vi "Convert Relative to Absolute Project Paths.vi"(9 "VI Relative Paths":string[](array[string]), 10 "Project File":path) -> (2 "VI Absolute Paths":path[](array[path]))   [LabVIEW 2011, in "VITesterUtilities.lvlib"]
uses:
  Libraries/VITesterUtilities.lvlib
  <userlib>/_OpenG.lib/file/file.llb/Build Path - File Names Array - path__ogtk.vi
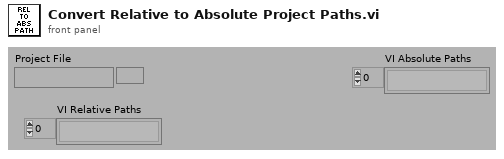
[diagram p1: front panel]
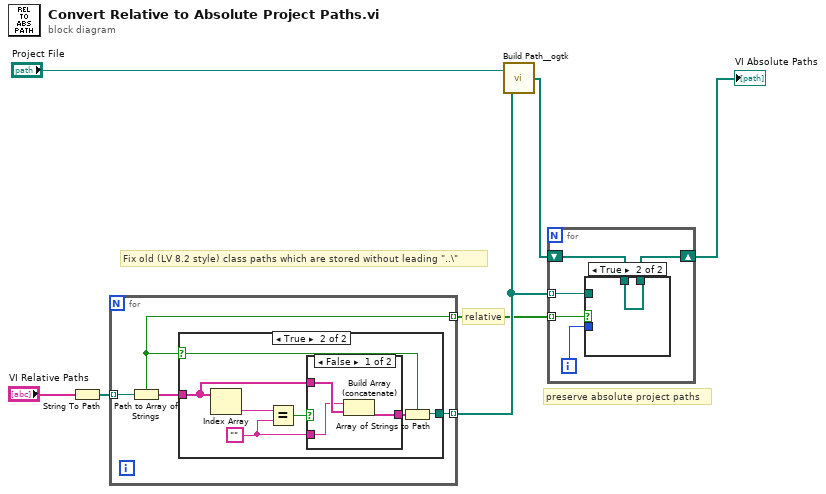
[diagram p0: block diagram]
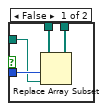
[diagram p2: hidden frame]
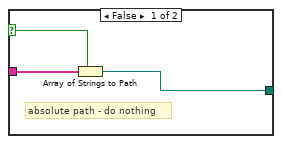
[diagram p3: hidden frame]
diagram:
  # "Fix old (LV 8.2 style) class paths which are stored without leading \"..\\\""
  # "preserve absolute project paths"
  # "relative"
  n1 = String To Path(string="VI Relative Paths") -> (path=w3:path[])
  n2 = for {
    tunnel: w3 -> [w11] mode=indexing
    tunnel: [w9] -> w7 mode=indexing
    tunnel: [w8] -> w4 mode=indexing
    n3 = Path to Array of Strings(0:w11) -> (1:w8:bool, 2:w10:string[])
    n4 = case shown="True" w8 {
      selector: w8 -> [w14 w16]
      tunnel: w10 -> [w13 w19]
      tunnel: [w12 w18] -> w9
      frame False {
        # "absolute path - do nothing"
        n5 = Array of Strings to Path(0:w13, 1:w14) -> (2:w12:path)
      }
      frame True {
        w15 = ""
        n6 = Index Array(array=w19) -> (element=w21:string)  [unwired: 1 in]
        n7 = Equal?(x=w21, y=w15) -> (x = y?=w20:bool)
        n8 = case shown="False" w20 {
          tunnel: w19 -> [w24 w25]
          tunnel: w15 -> [w23 _]
          tunnel: [w22 w25] -> w17
          frame False {
            n9 = Build Array (concatenate)(w23, w24) -> (w22:string[])
          }
          frame True {
          }
        }
        n10 = Array of Strings to Path(0:w17, 1:w16) -> (2:w18:path)
      }
    }
  }
  n11 = call-poly <userlib>:"Build Path__ogtk.vi"("name or relative path"=w7, "base path"="Project File") -> ("appended path"=w5:path[])
  n12 = for {
    tunnel: w4 -> [w26] mode=indexing
    shift-right: [w28] -> w6
    shift-left: w5 -> [w29]
    tunnel: w7 -> [w27] mode=indexing
    i -> [w30]
    n13 = case shown="True" w26 {
      tunnel: w30 -> [w34 _]
      tunnel: w29 -> [w33 w35]
      tunnel: [w32 w35] -> w28
      tunnel: w27 -> [w31 _]
      frame False {
        n14 = Replace Array Subset(array=w33, new element=w31, index=w34) -> (w32:path[])
      }
      frame True {
      }
    }
  }
  "VI Absolute Paths" <- w6
